vi "Normalize and Deadband.vi"(11 "Numeric in":dbl) -> (3 "Numeric out":dbl)   [LabVIEW 2018]
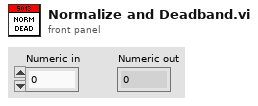
[diagram p1: front panel]
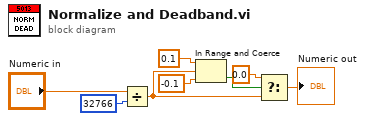
[diagram p0: block diagram]
diagram:
  n1 = Divide(x="Numeric in", y=32766) -> (x/y=w2:dbl)
  n2 = In Range and Coerce(upper limit=0.1, x=w2, lower limit=-0.1) -> (In Range?=w3:bool)  [unwired: 1 out]
  n3 = Select(t=0.0, s=w3, f=w2) -> (s? t:f=→"Numeric out":dbl)
